vi "Write File.vi"(8 "error in (no error)":errorcluster, 11 "Setup File in":refnum<class "Setup File.lvclass">) -> (0 "error out":errorcluster, 3 "Setup File out":refnum<class "Setup File.lvclass">)   [LabVIEW 2018, in "Setup File.lvclass"]
doc: "Este VI escreve em um arquivo texto a configuração contida na classe."
uses:
  Setup File.lvclass
  Setup File.lvclass/Setup File.ctl
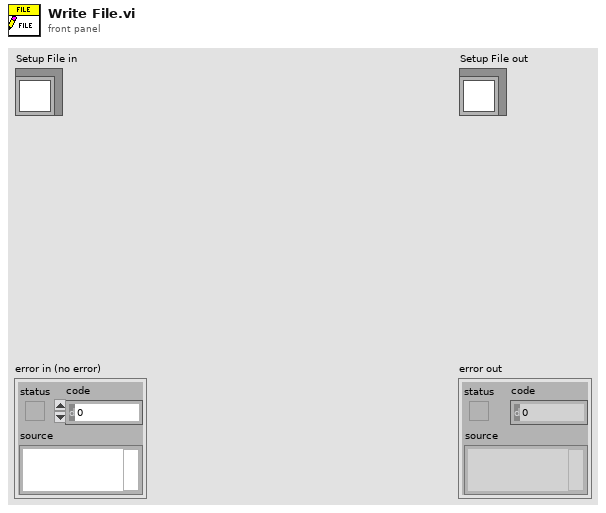
[diagram p1: front panel]
types:
  T1 = enum16{"open", "replace", "create", "open or create", "replace or create", "replace or create with confirmation"}
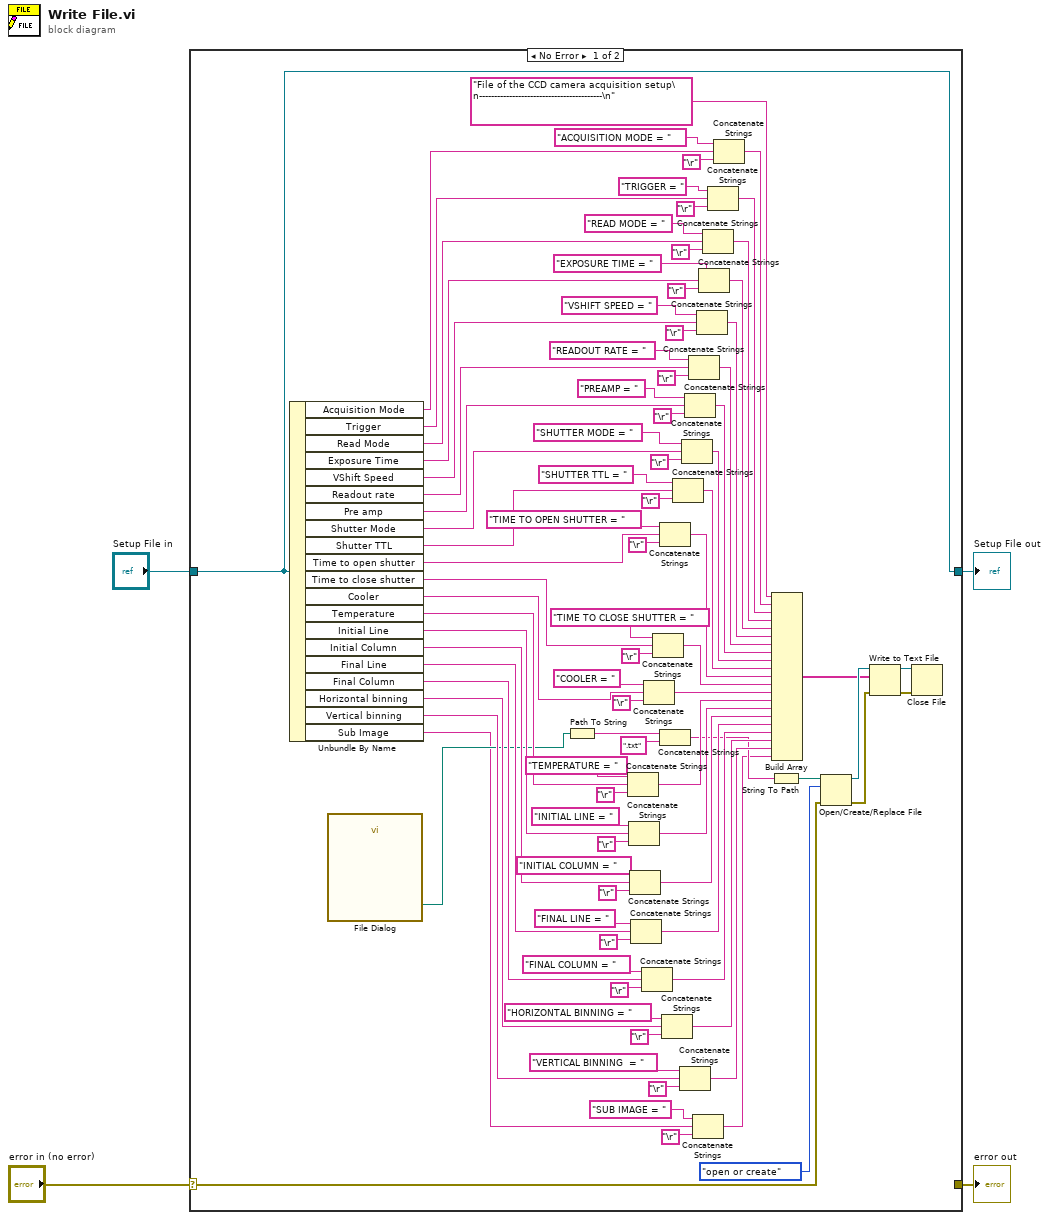
[diagram p0: block diagram]
diagram:
  n1 = case shown="No Error" "error in (no error)" {
    selector: "error in (no error)" -> [w93 w100]
    tunnel: [_ w100] -> w3
    tunnel: "Setup File in" -> [w55 w99]
    tunnel: [w55 w99] -> w1
    frame No Error {
      n2 = Unbundle By Name(w55) -> ("Acquisition Mode"=w91:string, "Trigger"=w89:string, "Read Mode"=w87:string, "Exposure Time"=w85:string, "VShift Speed"=w83:string, "Readout rate"=w81:string, "Pre amp"=w79:string, "Shutter Mode"=w77:string, "Shutter TTL"=w76:string, "Time to open shutter"=w74:string, "Time to close shutter"=w72:string, "Cooler"=w70:string, "Temperature"=w68:string, "Initial Line"=w66:string, "Initial Column"=w64:string, "Final Line"=w62:string, "Final Column"=w60:string, "Horizontal binning"=w57:string, "Vertical binning"=w56:string, "Sub Image"=w27:string)
      n3 = call "File Dialog"() -> ("selected path"=w33:path)  [unwired: 12 in, 3 out]
      n4 = Path To String(path=w33) -> (string=w32:string)
      n5 = Concatenate Strings("TEMPERATURE = ", w68, "\r") -> (w41:string)
      n6 = Concatenate Strings("INITIAL LINE = ", w66, "\r") -> (w40:string)
      n7 = Concatenate Strings("INITIAL COLUMN = ", w64, "\r") -> (w39:string)
      n8 = Concatenate Strings("FINAL LINE = ", w62, "\r") -> (w38:string)
      n9 = Concatenate Strings("FINAL COLUMN = ", w60, "\r") -> (w37:string)
      n10 = Concatenate Strings("COOLER = ", w70, "\r") -> (w42:string)
      n11 = Concatenate Strings("TIME TO CLOSE SHUTTER = ", w72, "\r") -> (w43:string)
      n12 = Concatenate Strings("TIME TO OPEN SHUTTER = ", w74, "\r") -> (w44:string)
      n13 = Concatenate Strings(w32, ".txt") -> (w30:string)
      n14 = Concatenate Strings("HORIZONTAL BINNING = ", w57, "\r") -> (w36:string)
      n15 = Concatenate Strings("SHUTTER TTL = ", w76, "\r") -> (w45:string)
      n16 = Concatenate Strings("VERTICAL BINNING  = ", w56, "\r") -> (w35:string)
      n17 = Concatenate Strings("SHUTTER MODE = ", w77, "\r") -> (w46:string)
      n18 = Concatenate Strings("PREAMP = ", w79, "\r") -> (w47:string)
      n19 = Concatenate Strings("READOUT RATE = ", w81, "\r") -> (w48:string)
      n20 = Concatenate Strings("SUB IMAGE = ", w27, "\r") -> (w26:string)
      n21 = Concatenate Strings("VSHIFT SPEED = ", w83, "\r") -> (w49:string)
      n22 = Concatenate Strings("EXPOSURE TIME = ", w85, "\r") -> (w50:string)
      n23 = Concatenate Strings("READ MODE = ", w87, "\r") -> (w51:string)
      n24 = Concatenate Strings("TRIGGER = ", w89, "\r") -> (w52:string)
      n25 = Concatenate Strings("ACQUISITION MODE = ", w91, "\r") -> (w53:string)
      n26 = String To Path(string=w30) -> (path=w29:path)
      n27 = Build Array("File of the CCD camera acquisition setup\n-----------------------------------------\n" ("string"), w53, w52, w51, w50, w49, w48, w47, w46, w45, w44, w43, w42, w41, w40, w39, w38, w37, w36, w35, w26) -> (w34:string[])
      n28 = Open/Create/Replace File(file path (use dialog)=w29, error in=w93, operation (0:open)=T1."open or create") -> (refnum out=w96:refnum<file>, error out=w98:errorcluster)  [unwired: 3 in, 1 out]
      n29 = Write to Text File(file (use dialog)=w96, text=w34, error in=w98) -> (refnum out=w95:refnum<file>, error out=w97:errorcluster)  [unwired: 1 in, 1 out]
      n30 = Close File(refnum=w95, error in=w97) -> ()  [unwired: 2 out]
    }
    frame Error {
    }
  }
  "error out" <- w3
  "Setup File out" <- w1
